vi "DDSCalibration.vi"() -> ()   [LabVIEW 2016]
panel:
  in  "appended array 2":dbl[](array[numeric])
  out "Waveform Chart":dbl[](graph)
  out "size(s) 13":i32
  out "appended array":dbl[](array[numeric])
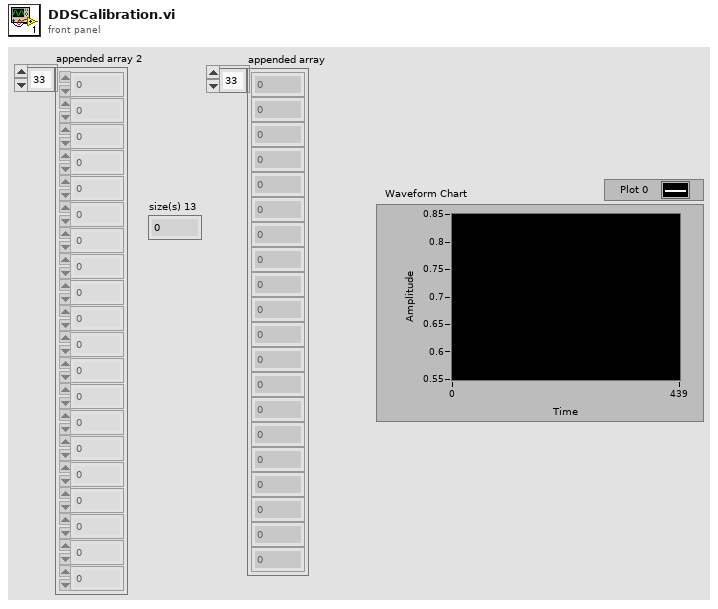
[diagram p1: front panel]
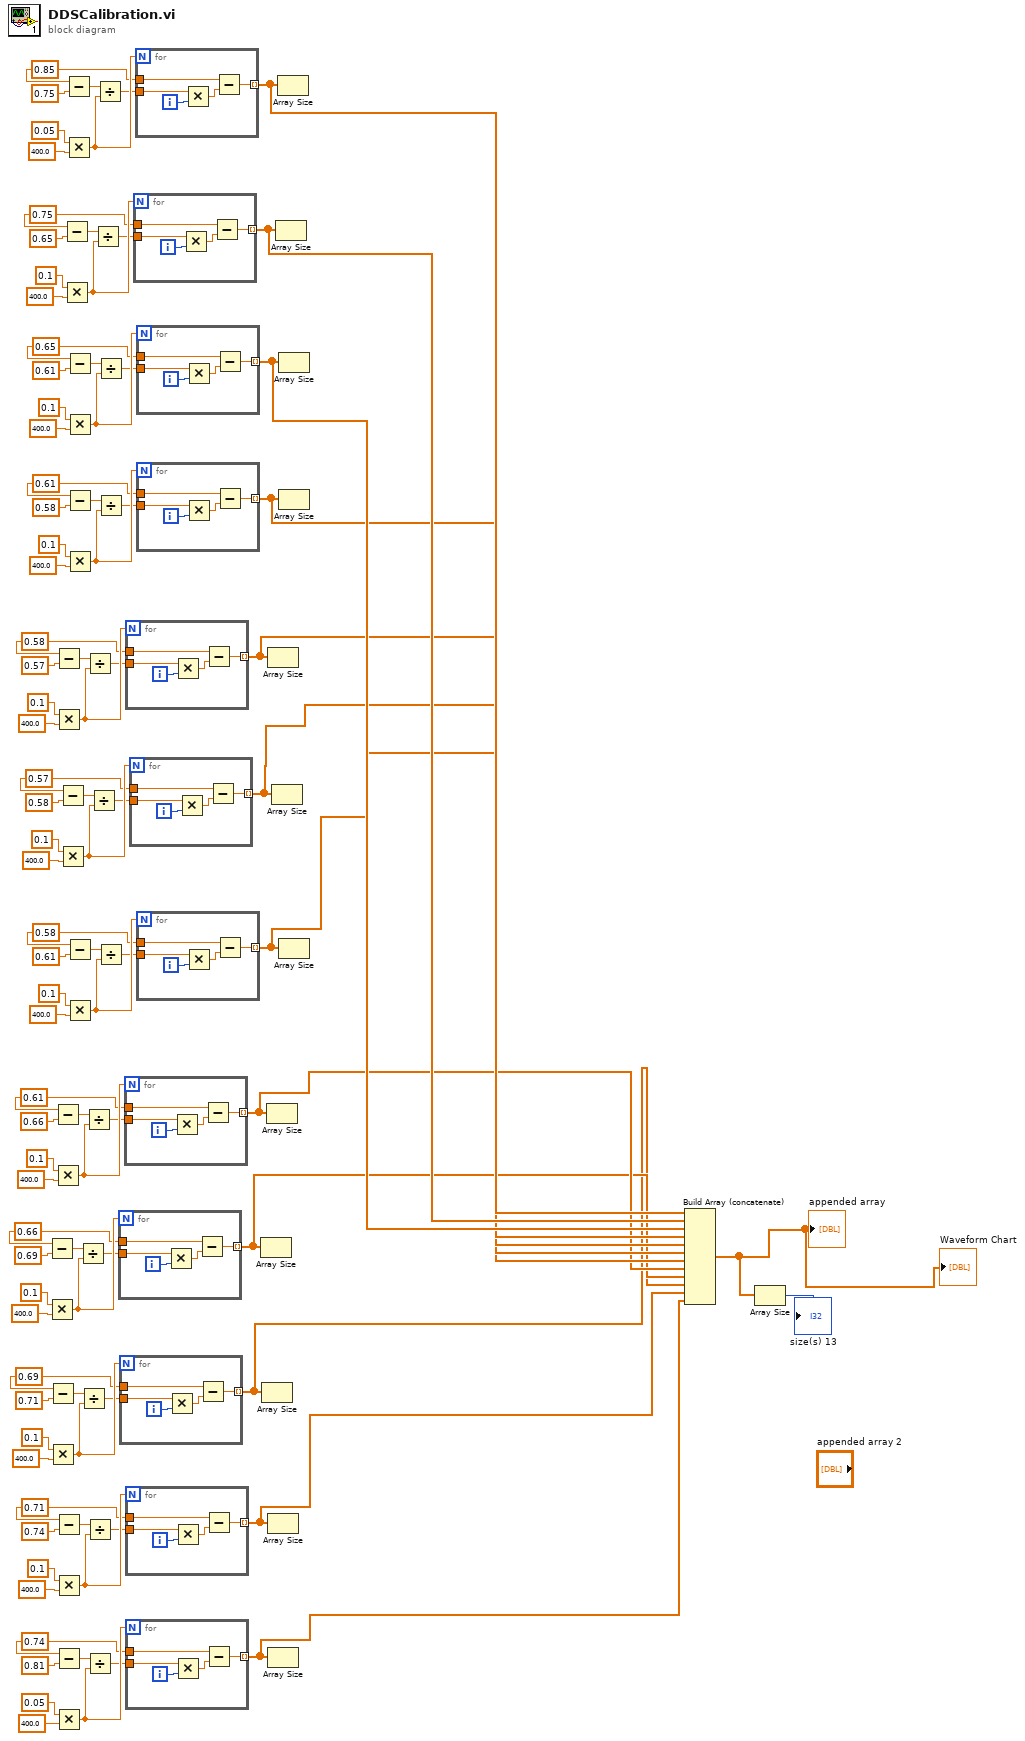
[diagram p0: block diagram]
diagram:
  w16 = 0.74 ("x")
  w23 = 0.71 ("x")
  w30 = 0.69 ("x")
  w37 = 0.66 ("x")
  w44 = 0.61 ("x")
  w51 = 0.58 ("x")
  w58 = 0.57 ("x")
  w65 = 0.58 ("x")
  w72 = 0.61 ("x")
  w79 = 0.65 ("x")
  w86 = 0.75 ("x")
  w93 = 0.85 ("x")
  n1 = Subtract(x=w37, y=0.69) -> (x-y=w39:dbl)
  n2 = Multiply(x=0.1, y=400.0) -> (x*y=w38:dbl)
  n3 = Subtract(x=w30, y=0.71) -> (x-y=w32:dbl)
  n4 = Multiply(x=0.1, y=400.0) -> (x*y=w31:dbl)
  n5 = Subtract(x=w44, y=0.66) -> (x-y=w46:dbl)
  n6 = Multiply(x=0.1, y=400.0) -> (x*y=w45:dbl)
  n7 = Subtract(x=w65, y=0.57) -> (x-y=w67:dbl)
  n8 = Multiply(x=0.1, y=400.0) -> (x*y=w66:dbl)
  n9 = Subtract(x=w23, y=0.74) -> (x-y=w25:dbl)
  n10 = Multiply(x=0.1, y=400.0) -> (x*y=w24:dbl)
  n11 = Subtract(x=w16, y=0.81) -> (x-y=w18:dbl)
  n12 = Multiply(x=0.05, y=400.0) -> (x*y=w17:dbl)
  n13 = Subtract(x=w58, y=0.58) -> (x-y=w60:dbl)
  n14 = Multiply(x=0.1, y=400.0) -> (x*y=w59:dbl)
  n15 = Subtract(x=w86, y=0.65) -> (x-y=w88:dbl)
  n16 = Multiply(x=0.1, y=400.0) -> (x*y=w87:dbl)
  n17 = Subtract(x=w93, y=0.75) -> (x-y=w95:dbl)
  n18 = Multiply(x=0.05, y=400.0) -> (x*y=w94:dbl)
  n19 = Subtract(x=w79, y=0.61) -> (x-y=w81:dbl)
  n20 = Multiply(x=0.1, y=400.0) -> (x*y=w80:dbl)
  n21 = Subtract(x=w72, y=0.58) -> (x-y=w74:dbl)
  n22 = Multiply(x=0.1, y=400.0) -> (x*y=w73:dbl)
  n23 = Subtract(x=w51, y=0.61) -> (x-y=w53:dbl)
  n24 = Multiply(x=0.1, y=400.0) -> (x*y=w52:dbl)
  n25 = Divide(x=w39, y=w38) -> (x/y=w36:dbl)
  n26 = Divide(x=w32, y=w31) -> (x/y=w29:dbl)
  n27 = Divide(x=w46, y=w45) -> (x/y=w43:dbl)
  n28 = Divide(x=w67, y=w66) -> (x/y=w64:dbl)
  n29 = Divide(x=w25, y=w24) -> (x/y=w22:dbl)
  n30 = Divide(x=w18, y=w17) -> (x/y=w15:dbl)
  n31 = Divide(x=w60, y=w59) -> (x/y=w57:dbl)
  n32 = Divide(x=w88, y=w87) -> (x/y=w85:dbl)
  n33 = Divide(x=w95, y=w94) -> (x/y=w92:dbl)
  n34 = Divide(x=w81, y=w80) -> (x/y=w78:dbl)
  n35 = Divide(x=w74, y=w73) -> (x/y=w71:dbl)
  n36 = Divide(x=w53, y=w52) -> (x/y=w50:dbl)
  n37 = for {
    N: w38 -> [_]
    tunnel: w37 -> [w103]
    tunnel: w36 -> [w101]
    tunnel: [w99] -> w6 mode=indexing
    i -> [w102]
    n38 = Multiply(x=w101, y=w102) -> (x*y=w100:dbl)
    n39 = Subtract(x=w103, y=w100) -> (x-y=w99:dbl)
  }
  n40 = for {
    N: w31 -> [_]
    tunnel: w30 -> [w108]
    tunnel: w29 -> [w106]
    tunnel: [w104] -> w5 mode=indexing
    i -> [w107]
    n41 = Multiply(x=w106, y=w107) -> (x*y=w105:dbl)
    n42 = Subtract(x=w108, y=w105) -> (x-y=w104:dbl)
  }
  n43 = for {
    N: w45 -> [_]
    tunnel: w44 -> [w113]
    tunnel: w43 -> [w111]
    tunnel: [w109] -> w7 mode=indexing
    i -> [w112]
    n44 = Multiply(x=w111, y=w112) -> (x*y=w110:dbl)
    n45 = Subtract(x=w113, y=w110) -> (x-y=w109:dbl)
  }
  n46 = for {
    N: w66 -> [_]
    tunnel: w65 -> [w118]
    tunnel: w64 -> [w116]
    tunnel: [w114] -> w10 mode=indexing
    i -> [w117]
    n47 = Multiply(x=w116, y=w117) -> (x*y=w115:dbl)
    n48 = Subtract(x=w118, y=w115) -> (x-y=w114:dbl)
  }
  n49 = for {
    N: w24 -> [_]
    tunnel: w23 -> [w123]
    tunnel: w22 -> [w121]
    tunnel: [w119] -> w4 mode=indexing
    i -> [w122]
    n50 = Multiply(x=w121, y=w122) -> (x*y=w120:dbl)
    n51 = Subtract(x=w123, y=w120) -> (x-y=w119:dbl)
  }
  n52 = for {
    N: w17 -> [_]
    tunnel: w16 -> [w128]
    tunnel: w15 -> [w126]
    tunnel: [w124] -> w3 mode=indexing
    i -> [w127]
    n53 = Multiply(x=w126, y=w127) -> (x*y=w125:dbl)
    n54 = Subtract(x=w128, y=w125) -> (x-y=w124:dbl)
  }
  n55 = for {
    N: w59 -> [_]
    tunnel: w58 -> [w133]
    tunnel: w57 -> [w131]
    tunnel: [w129] -> w9 mode=indexing
    i -> [w132]
    n56 = Multiply(x=w131, y=w132) -> (x*y=w130:dbl)
    n57 = Subtract(x=w133, y=w130) -> (x-y=w129:dbl)
  }
  n58 = for {
    N: w87 -> [_]
    tunnel: w86 -> [w138]
    tunnel: w85 -> [w136]
    tunnel: [w134] -> w13 mode=indexing
    i -> [w137]
    n59 = Multiply(x=w136, y=w137) -> (x*y=w135:dbl)
    n60 = Subtract(x=w138, y=w135) -> (x-y=w134:dbl)
  }
  n61 = for {
    N: w94 -> [_]
    tunnel: w93 -> [w143]
    tunnel: w92 -> [w141]
    tunnel: [w139] -> w14 mode=indexing
    i -> [w142]
    n62 = Multiply(x=w141, y=w142) -> (x*y=w140:dbl)
    n63 = Subtract(x=w143, y=w140) -> (x-y=w139:dbl)
  }
  n64 = for {
    N: w80 -> [_]
    tunnel: w79 -> [w148]
    tunnel: w78 -> [w146]
    tunnel: [w144] -> w12 mode=indexing
    i -> [w147]
    n65 = Multiply(x=w146, y=w147) -> (x*y=w145:dbl)
    n66 = Subtract(x=w148, y=w145) -> (x-y=w144:dbl)
  }
  n67 = for {
    N: w73 -> [_]
    tunnel: w72 -> [w153]
    tunnel: w71 -> [w151]
    tunnel: [w149] -> w11 mode=indexing
    i -> [w152]
    n68 = Multiply(x=w151, y=w152) -> (x*y=w150:dbl)
    n69 = Subtract(x=w153, y=w150) -> (x-y=w149:dbl)
  }
  n70 = for {
    N: w52 -> [_]
    tunnel: w51 -> [w158]
    tunnel: w50 -> [w156]
    tunnel: [w154] -> w8 mode=indexing
    i -> [w157]
    n71 = Multiply(x=w156, y=w157) -> (x*y=w155:dbl)
    n72 = Subtract(x=w158, y=w155) -> (x-y=w154:dbl)
  }
  n73 = Array Size(array=w6) -> ()  [unwired: 1 out]
  n74 = Array Size(array=w5) -> ()  [unwired: 1 out]
  n75 = Array Size(array=w7) -> ()  [unwired: 1 out]
  n76 = Array Size(array=w10) -> ()  [unwired: 1 out]
  n77 = Array Size(array=w4) -> ()  [unwired: 1 out]
  n78 = Array Size(array=w3) -> ()  [unwired: 1 out]
  n79 = Array Size(array=w9) -> ()  [unwired: 1 out]
  n80 = Array Size(array=w13) -> ()  [unwired: 1 out]
  n81 = Array Size(array=w14) -> ()  [unwired: 1 out]
  n82 = Array Size(array=w12) -> ()  [unwired: 1 out]
  n83 = Array Size(array=w11) -> ()  [unwired: 1 out]
  n84 = Array Size(array=w8) -> ()  [unwired: 1 out]
  n85 = Build Array (concatenate)(w14, w13, w12, w11, w10, w9, w8, w7, w6, w5, w4, w3) -> (w1:dbl[])
  "appended array" <- w1
  "Waveform Chart" <- w1
  n86 = Array Size(array=w1) -> (size(s)=→"size(s) 13":i32)
